vi "arrayplot.vi"() -> ()   [LabVIEW 2022 SP3]
uses:
  <vilib>/numeric/Random Number (Range) U64.vi
  <vilib>/numeric/sub_Random U32.vi
panel:
  out "Waveform Graph 2":u64[][](graph)
  out "Waveform Graph":cluster{u64[]}[](graph)
  out "20 values":dbl[](array[numeric])
  out "15 values":dbl[](array[numeric])
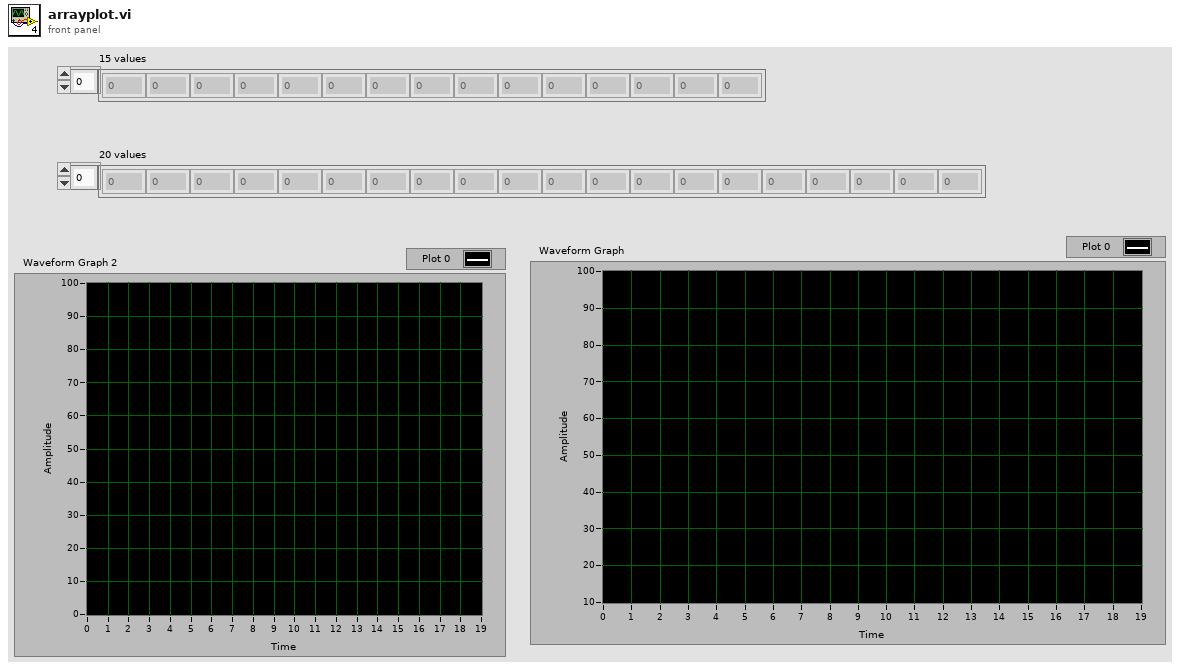
[diagram p1: front panel]
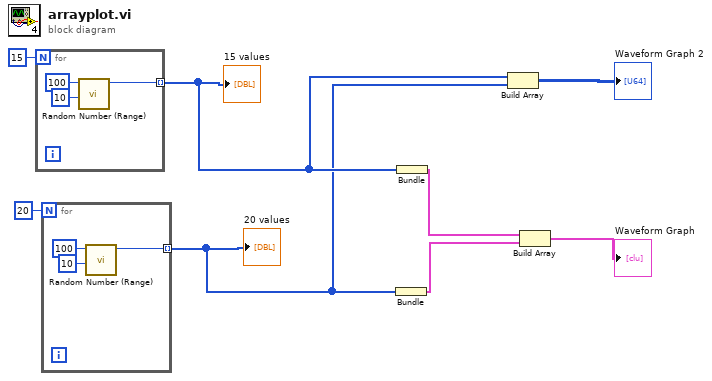
[diagram p0: block diagram]
diagram:
  n1 = for {
    N: 15 -> [_]
    tunnel: [w9] -> w3 mode=indexing
    n2 = call-poly <vilib>:"Random Number (Range).vi"("lower bound (0)"=u64 10, "upper bound (100)"=u64 100) -> ("number"=w9:u64)  [unwired: 9 in]
  }
  "15 values" <- w3
  n3 = for {
    N: 20 -> [_]
    tunnel: [w12] -> w2 mode=indexing
    n4 = call-poly <vilib>:"Random Number (Range).vi"("lower bound (0)"=u64 10, "upper bound (100)"=u64 100) -> ("number"=w12:u64)  [unwired: 9 in]
  }
  "20 values" <- w2
  n5 = Bundle "Bundle"(w2) -> (w5:cluster{u64[]})  [unwired: 1 in]
  n6 = Bundle "Bundle"(w3) -> (w6:cluster{u64[]})  [unwired: 1 in]
  n7 = Build Array(w3, w2) -> (→"Waveform Graph 2":u64[][])
  n8 = Build Array(w6, w5) -> (→"Waveform Graph":cluster{u64[]}[])
